vi "String - Create [LayoutFileName].vi"(9 "2014-11-07 15:18\nMaster Data Layout":T1[](array[typedef]), 10 "[PlantId]":string, 11 "MCListBox Row Data":string[](array[string])) -> (3 "[LayoutFileName]":string)   [LabVIEW 2013]
uses:
  Controls/DB - Master Data Layout Enum.ctl
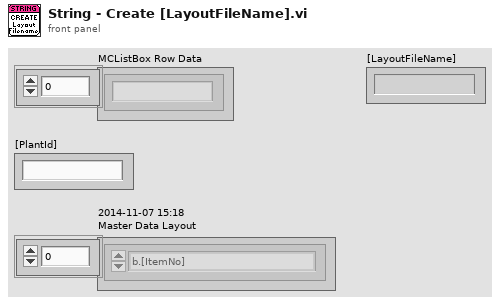
[diagram p1: front panel]
types:
  T1 = typedef "DB - Master Data Layout Enum.ctl" = enum16{"b.[ItemNo]", "a.[OutputSetId]", "a.[Description]", "a.[Default]", "a.[Inactive]", "b.[OutputTypeId]", "c.[ShortDescription]", "b.[Output]", "b.[Inactive]", "b.[LayoutId]", "b.[Description]", "b.[LayoutFileName]", "b.[LayoutFilePath]"}
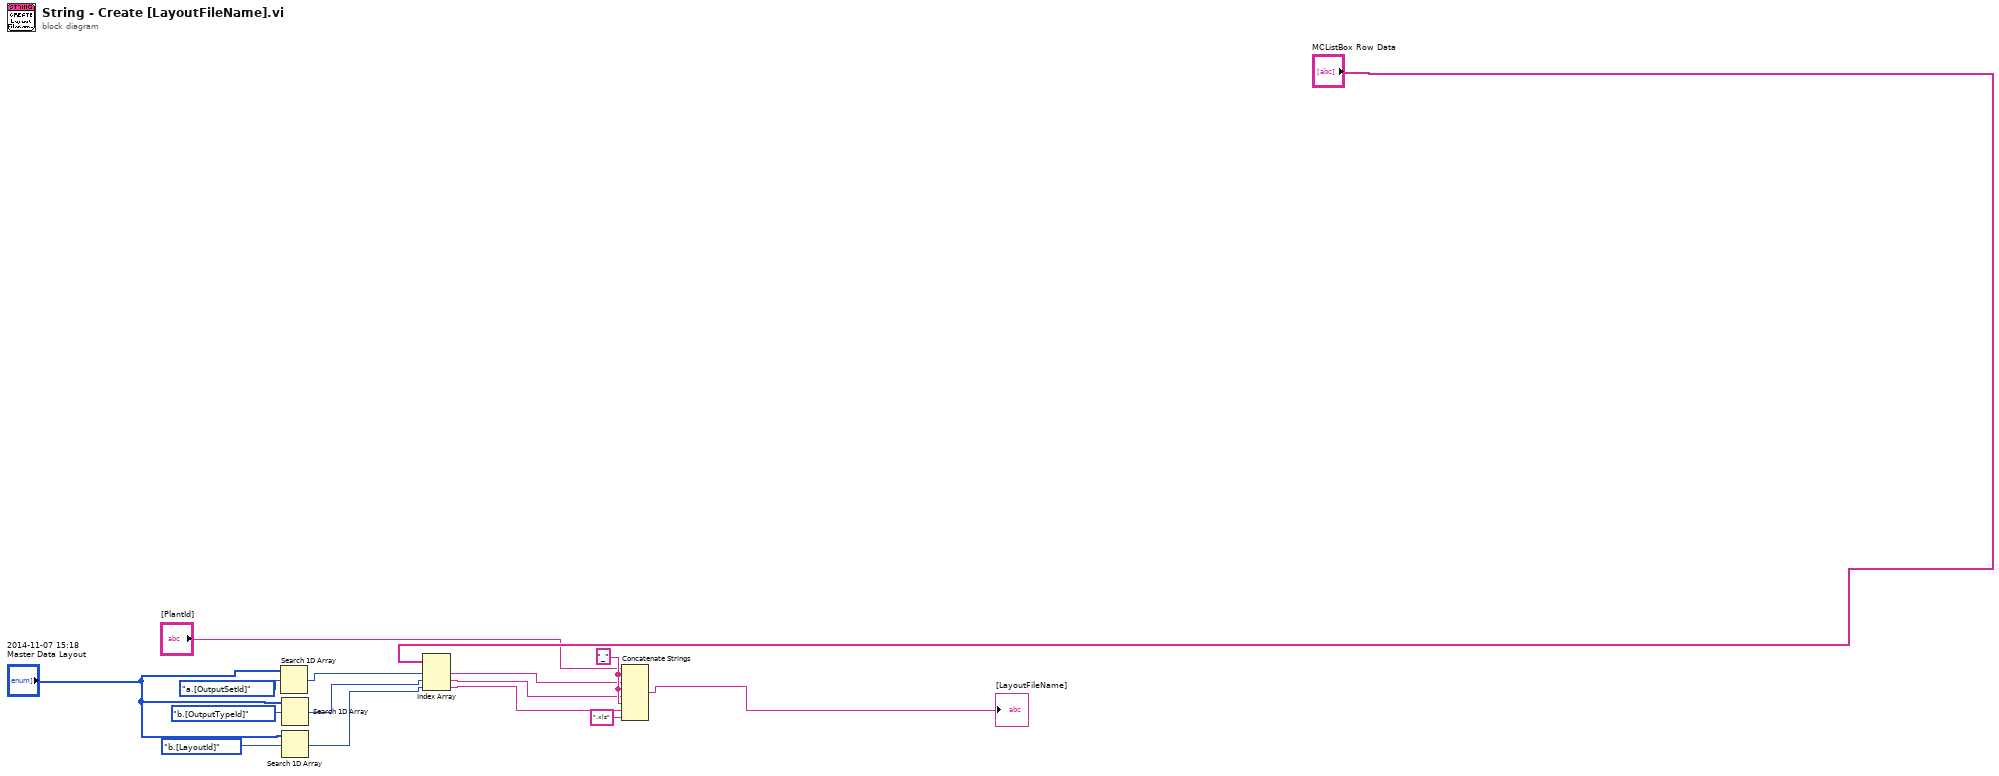
[diagram p0: block diagram]
diagram:
  w10 = "_"
  n1 = Search 1D Array(1D array="2014-11-07 15:18\nMaster Data Layout", element=DB_-_Master_Data_Layout_Enum."a.[OutputSetId]" ("2014-11-07 13:45\nMaster Data Layout")) -> (index of element=w2:i32)  [unwired: 1 in]
  n2 = Search 1D Array(1D array="2014-11-07 15:18\nMaster Data Layout", element=DB_-_Master_Data_Layout_Enum."b.[OutputTypeId]" ("2014-11-07 13:45\nMaster Data Layout")) -> (index of element=w5:i32)  [unwired: 1 in]
  n3 = Search 1D Array(1D array="2014-11-07 15:18\nMaster Data Layout", element=DB_-_Master_Data_Layout_Enum."b.[LayoutId]" ("2014-11-07 13:45\nMaster Data Layout")) -> (index of element=w6:i32)  [unwired: 1 in]
  n4 = Index Array(array="MCListBox Row Data", index #1=w2, index #2=w5, index #3=w6) -> (element #1=w8:string, element #2=w9:string, element #3=w11:string)
  n5 = Concatenate Strings("[PlantId]", w10, w8, w10, w9, w10, w11, ".xls" ("string")) -> (→"[LayoutFileName]":string)
